vi "Draw y=0 line.vi"(8 "Error":errorcluster, 9 "Waveform":waveform(dbl), 10 "State":T1={"Measure ?"=[], "Direction"=[], "Loop ?"={"Start"=0, "Finish"=2}, "Storage Location"=[], "Show Current Location"=FALSE, "Current Location"=0, "Show y=0"=FALSE, "Program"=[], "Index"=0, "Average During Loop ?"=FALSE, "# of Loops"=1, "Loop Control"={0, 2}, "Units"="", "Digits"=0, "Significant Figures (F) or DP (T)"=FALSE, "Rate Mode"=FALSE, "Current Y value"=0.0, "Initial Value"=0.0} {"# of Loops" min=1 step=1; "Index" min=0 step=1; "Program"."Step" min=0.001 max=80.0 step=0.001 format="%.2f"; "Program"."Target" format="%.2f"}, 11 "Plots":cluster{"X":dbl[], "Y":dbl[]}[](array[cluster])) -> (0 "Error Out":errorcluster, 3 "Plots Out":cluster{"X":dbl[], "Y":dbl[]}[](array[cluster]))   [LabVIEW 2018, in "Multi Segment Waveform.xctl"]
doc: "Generates a waveform that is NaN apart from the one point at the given index position. The Y value of this point is the same as the corresponding point in the first waveform of the array input,"
uses:
  Multi Segment Waveform.xctl
  State.ctl
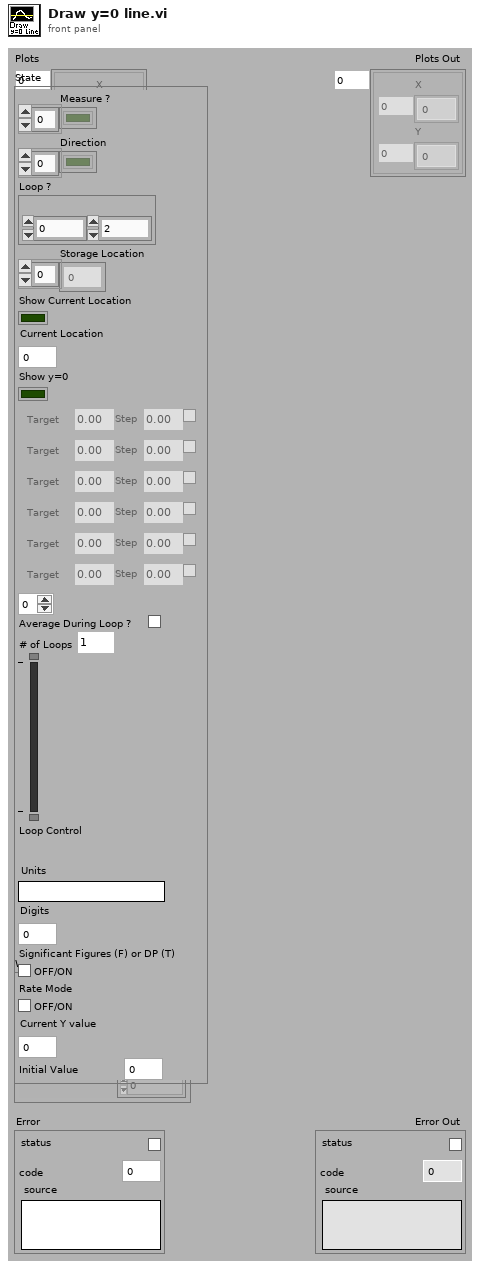
[diagram p1: front panel]
types:
  T1 = typedef "Multi Segment Waveform.xctl/State.ctl" = cluster{"Measure ?":bool[], "Direction":bool[], "Loop ?":cluster{"Start":i32, "Finish":i32}, "Storage Location":i32[], "Show Current Location":bool, "Current Location":i32, "Show y=0":bool, "Program":cluster{"Target":dbl, "Step":dbl, "Measure ?":bool}[], "Index":i32, "Average During Loop ?":bool, "# of Loops":u32, "Loop Control":cluster{i32, i32}, "Units":string, "Digits":i32, "Significant Figures (F) or DP (T)":bool, "Rate Mode":bool, "Current Y value":dbl, "Initial Value":dbl}
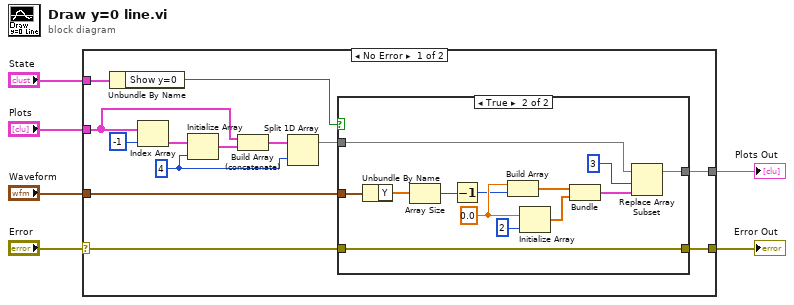
[diagram p0: block diagram]
diagram:
  n1 = case shown="No Error" "Error" {
    selector: "Error" -> [w15 w36]
    tunnel: "Plots" -> [w8 w35]
    tunnel: "State" -> [w19 _]
    tunnel: "Waveform" -> [w17 _]
    tunnel: [w16 w35] -> w3
    tunnel: [w14 w36] -> w1
    frame No Error {
      w13 = 4 ("dimension size")
      n2 = Unbundle By Name(w19) -> ("Show y=0"=w18:bool)
      n3 = Index Array(array=w8, index=-1) -> (element=w10:cluster{"X":dbl[], "Y":dbl[]})
      n4 = Initialize Array(w10, w13) -> (w11:cluster{"X":dbl[], "Y":dbl[]}[])
      n5 = Build Array (concatenate)(w8, w11) -> (w12:cluster{"X":dbl[], "Y":dbl[]}[])
      n6 = Split 1D Array(array=w12, index=w13) -> (first subarray=w7:cluster{"X":dbl[], "Y":dbl[]}[])  [unwired: 1 out]
      n7 = case shown="True" w18 {
        tunnel: w7 -> [w21 w33]
        tunnel: w17 -> [_ w25]
        tunnel: [w21 w30] -> w16
        tunnel: w15 -> [w20 w29]
        tunnel: [w20 w29] -> w14
        frame False {
        }
        frame True {
          w26 = 0.0 ("element")
          n8 = Unbundle By Name(w25) -> ("Y"=w24:dbl[])
          n9 = Array Size(array=w24) -> (size(s)=w23:i32)
          n10 = Decrement(x=w23) -> (x-1=w22:i32)
          n11 = Build Array(w26, w22) -> (w34:dbl[])
          n12 = Initialize Array(w26, 2 ("dimension size")) -> (w27:dbl[])
          n13 = Bundle(w34, w27) -> (w31:cluster{dbl[], dbl[]})  [unwired: 1 out]
          n14 = Replace Array Subset(array=w33, new element=w31, index=3) -> (w30:cluster{"X":dbl[], "Y":dbl[]}[])
        }
      }
    }
    frame Error {
    }
  }
  "Plots Out" <- w3
  "Error Out" <- w1
